vi "TEMPDo.vi"(8 "error in (no error)":errorcluster, 10 "Actor in":refnum<class "Actor.lvclass">, 11 "DNL_Message Template":refnum<class "Message.lvclass">) -> (0 "error out":errorcluster, 2 "Actor out":refnum<class "Actor.lvclass">)   [LabVIEW 2016, in "Return Template.lvclass"]
doc: "This VI delivers the message to the actor by calling the appropriate method(s) on the actor."
uses:
  Return Template.lvclass
  <vilib>/ActorFramework/Actor/Actor.lvclass
  <vilib>/ActorFramework/Message/Message.lvclass
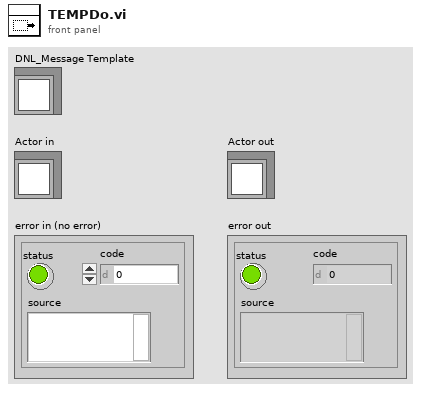
[diagram p1: front panel]
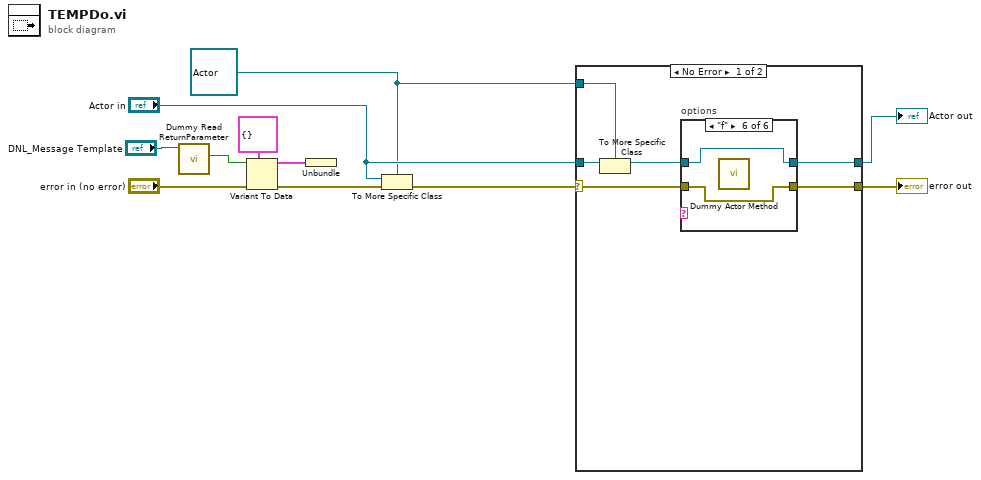
[diagram p0: block diagram]
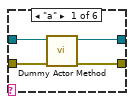
[diagram p2: hidden frame]
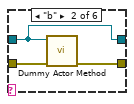
[diagram p3: hidden frame]
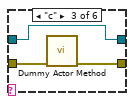
[diagram p4: hidden frame]
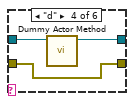
[diagram p5: hidden frame]
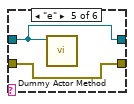
[diagram p6: hidden frame]
diagram:
  w7 = refnum<class "Actor.lvclass"> refnum ("Actor in")
  n1 = call "Dummy Read ReturnParameter.vi"("Actor in"="DNL_Message Template") -> ("Boolean"=w1:bool)  [unwired: 8 in, 2 out]
  n2 = Variant To Data(error in="error in (no error)", type=cluster{} {} ("Type"), Variant=w1) -> (data=w6:cluster{}, error out=w3:errorcluster)
  n3 = Unbundle ("Main-Unbundle")(w6) -> ()  [unwired: 1 out]
  n4 = To More Specific Class(target class=w7, reference="Actor in", error in=w3) -> (error out=w11:errorcluster)  [unwired: 1 out]
  n5 = case shown="No Error" w11 {
    selector: w11 -> [w15 w36]
    tunnel: [w17 w36] -> w10
    tunnel: [w16 w35] -> w9
    tunnel: "Actor in" -> [w14 w35]
    tunnel: w7 -> [w13 _]
    frame No Error {
      n6 = To More Specific Class(target class=w13, reference=w14) -> (specific class reference=w12:refnum<class "Actor.lvclass">)  [unwired: 1 in, 1 out]
      n7 = case "options" shown="\"f\"" {
        selector: _ -> [_ _ _ _ _ _]
        tunnel: [w21 w24 w27 w30 w31 w33] -> w17
        tunnel: [w20 w22 w25 w28 w32 w34] -> w16
        tunnel: w15 -> [w19 w23 w26 w30 w31 w33]
        tunnel: w12 -> [w18 w22 w25 w29 w32 w34]
        frame "a" {
          n8 = call "Dummy Actor Method.vi"("error in (no error)"=w19, "Actor in"=w18) -> ("error out"=w21:errorcluster, "Actor out"=w20:refnum<class "Actor.lvclass">)  [unwired: 8 in]
        }
        frame "b" {
          n9 = call "Dummy Actor Method.vi"("error in (no error)"=w23, "Actor in"=w22) -> ("error out"=w24:errorcluster)  [unwired: 8 in, 1 out]
        }
        frame "c" {
          n10 = call "Dummy Actor Method.vi"("error in (no error)"=w26) -> ("error out"=w27:errorcluster)  [unwired: 9 in, 1 out]
        }
        frame "d" {
          n11 = call "Dummy Actor Method.vi"("Actor in"=w29) -> ("Actor out"=w28:refnum<class "Actor.lvclass">)  [unwired: 9 in, 1 out]
        }
        frame "e" {
          n12 = call "Dummy Actor Method.vi"("Actor in"=w32) -> ()  [unwired: 9 in, 2 out]
        }
        frame "f" {
          n13 = call "Dummy Actor Method.vi"() -> ()  [unwired: 10 in, 2 out]
        }
      }
    }
    frame Error {
    }
  }
  "error out" <- w10
  "Actor out" <- w9
